vi "gnuplotVectors.vi"(4 "VectorFileLocation":path) -> (0 "Plot data file":path, 1 "gnuplotScript":string, 2 "Saved Automatically?":bool)   [LabVIEW 2013]
uses:
  Results_plotter_Global.vi
panel:
  in  "OpenLogfile?":bool
  in  "Show Script Editor?":bool
  in  "Tab Control":enum32{"OtherStuff ", "TerminalTest"}(tab)
  out "AuditTrail":string[](array[string])
  # "Shows the numbered line colours and point styles available- well it would, if it didn't disappear every time I update from the repository..!"
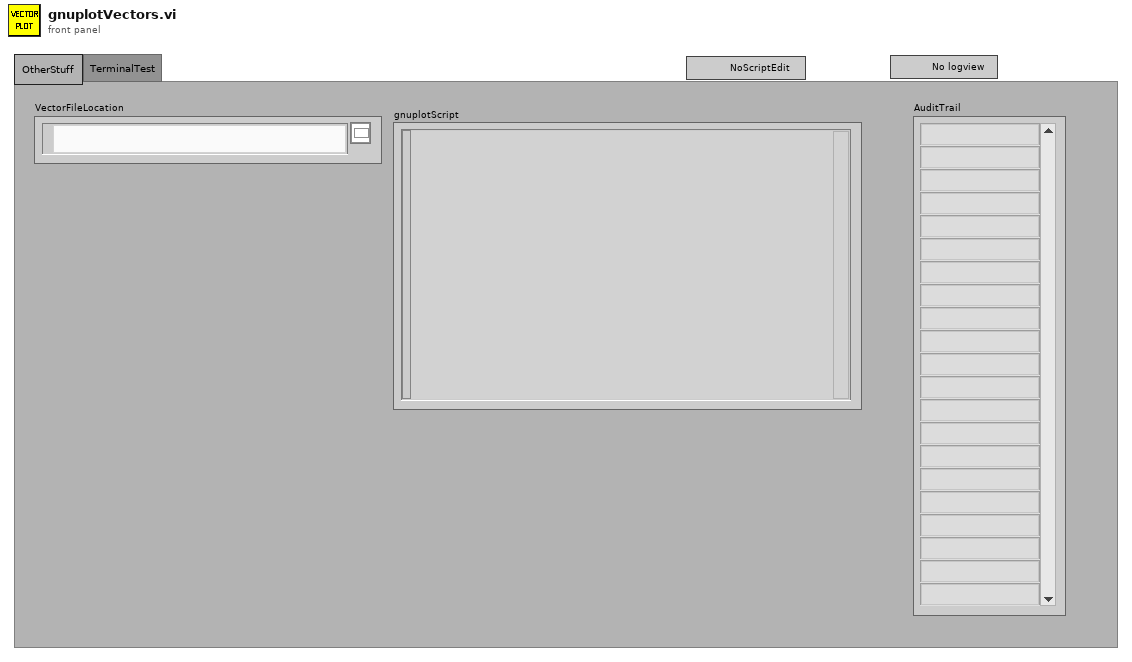
[diagram p1: front panel]
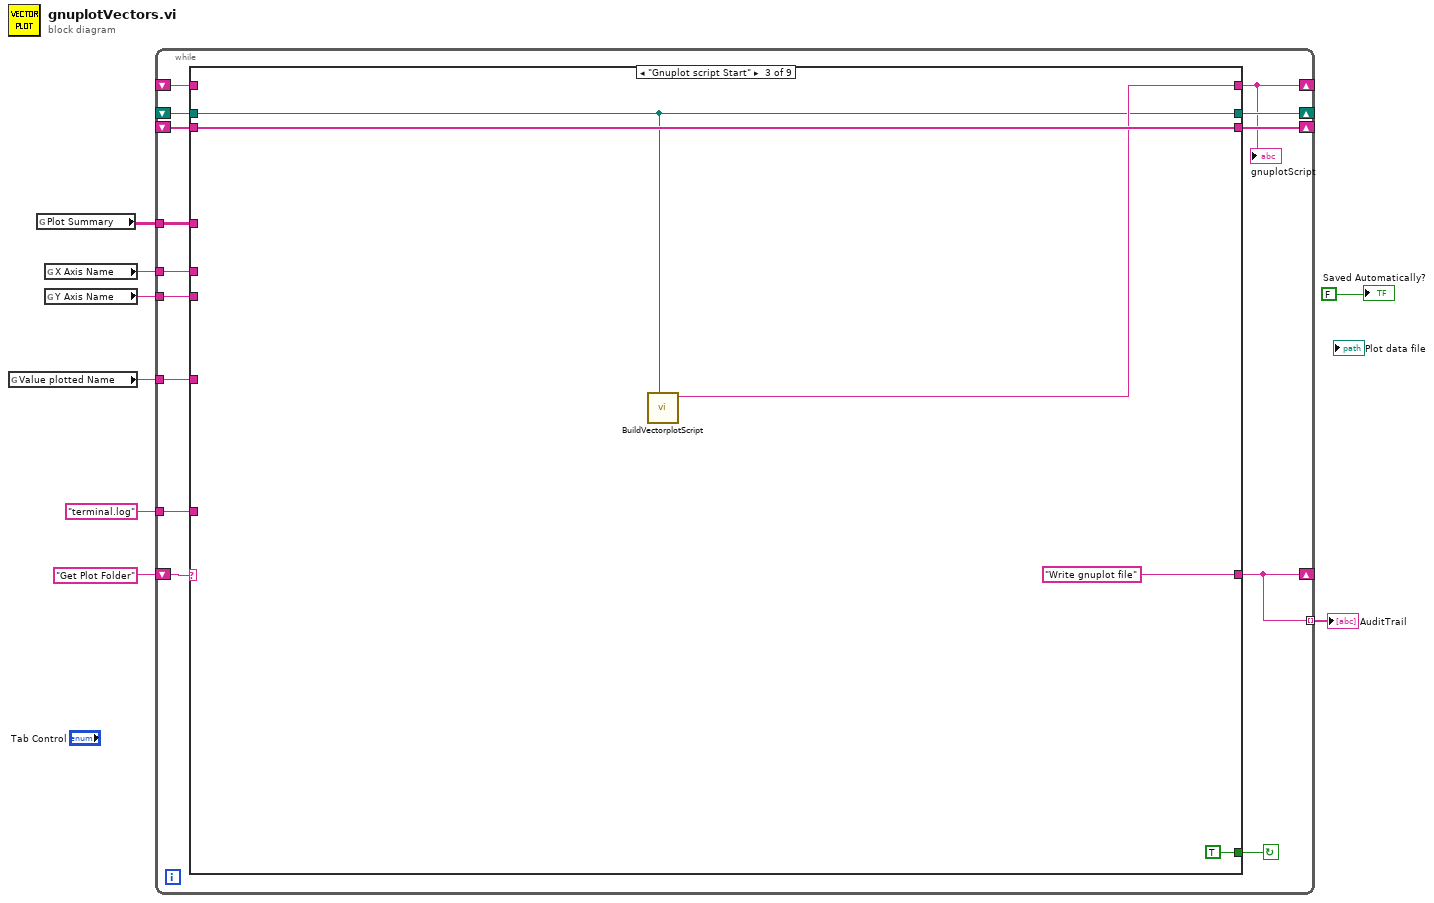
[diagram p0: block diagram]
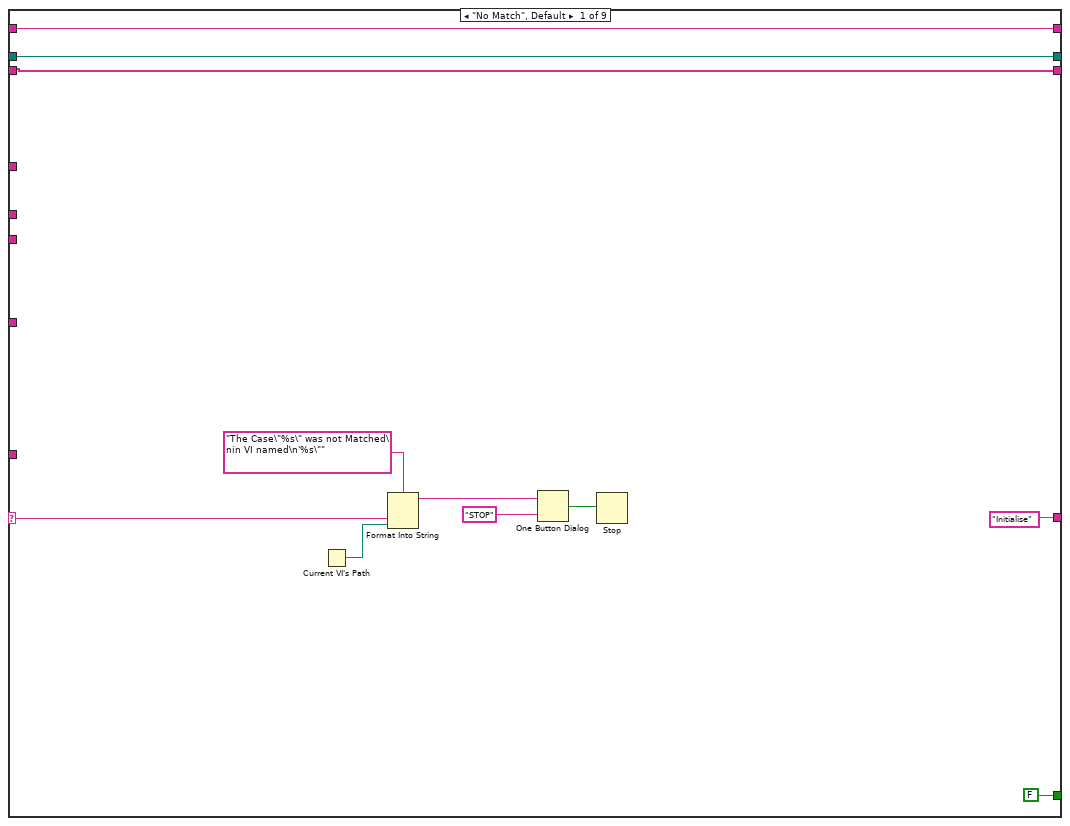
[diagram p2: hidden frame]
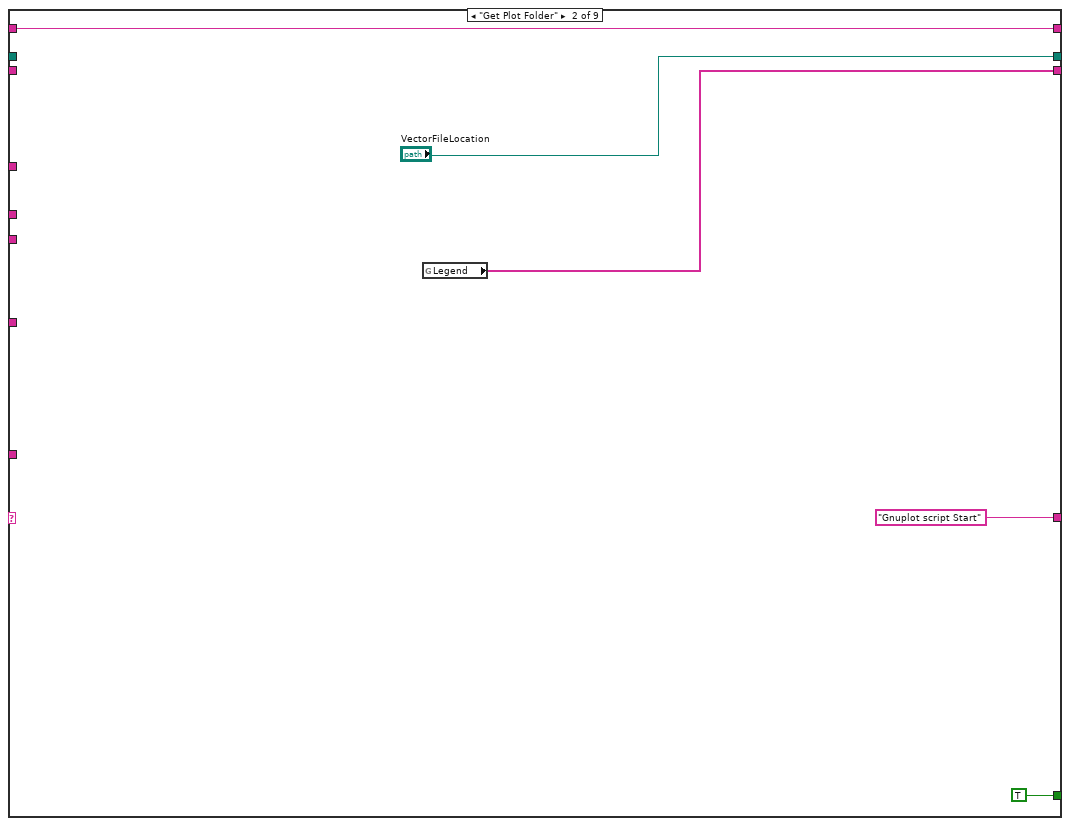
[diagram p3: hidden frame]
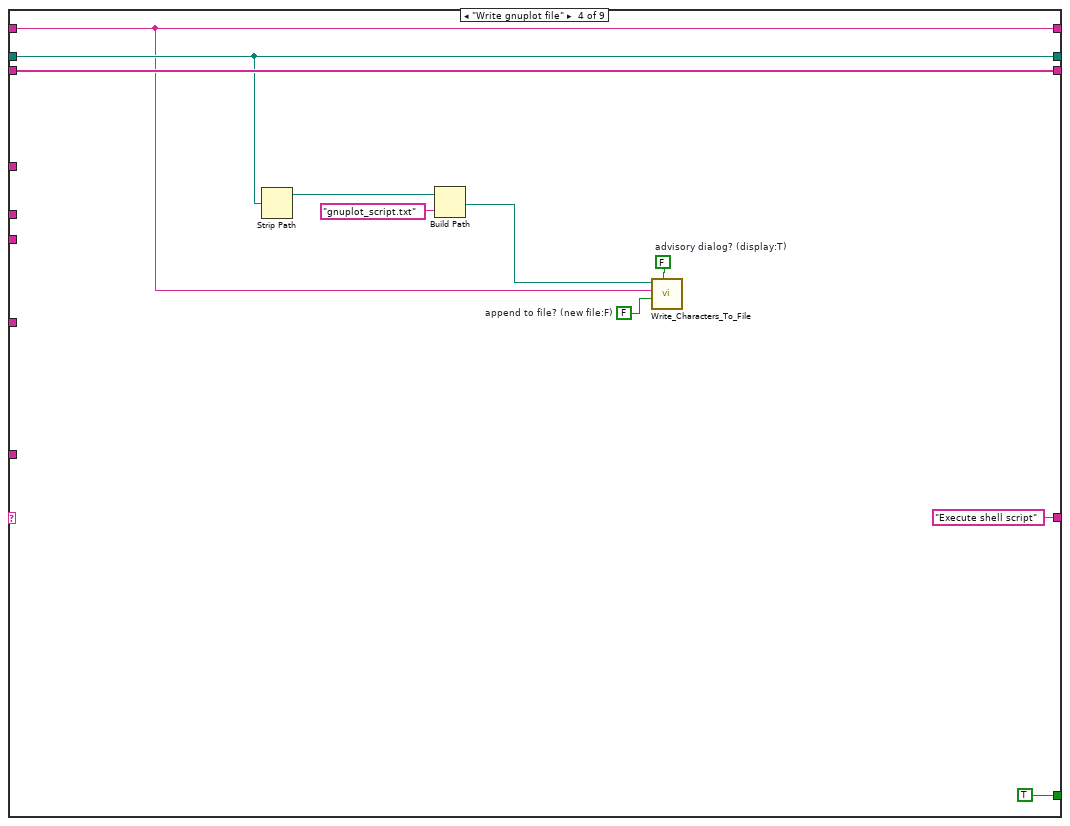
[diagram p4: hidden frame]
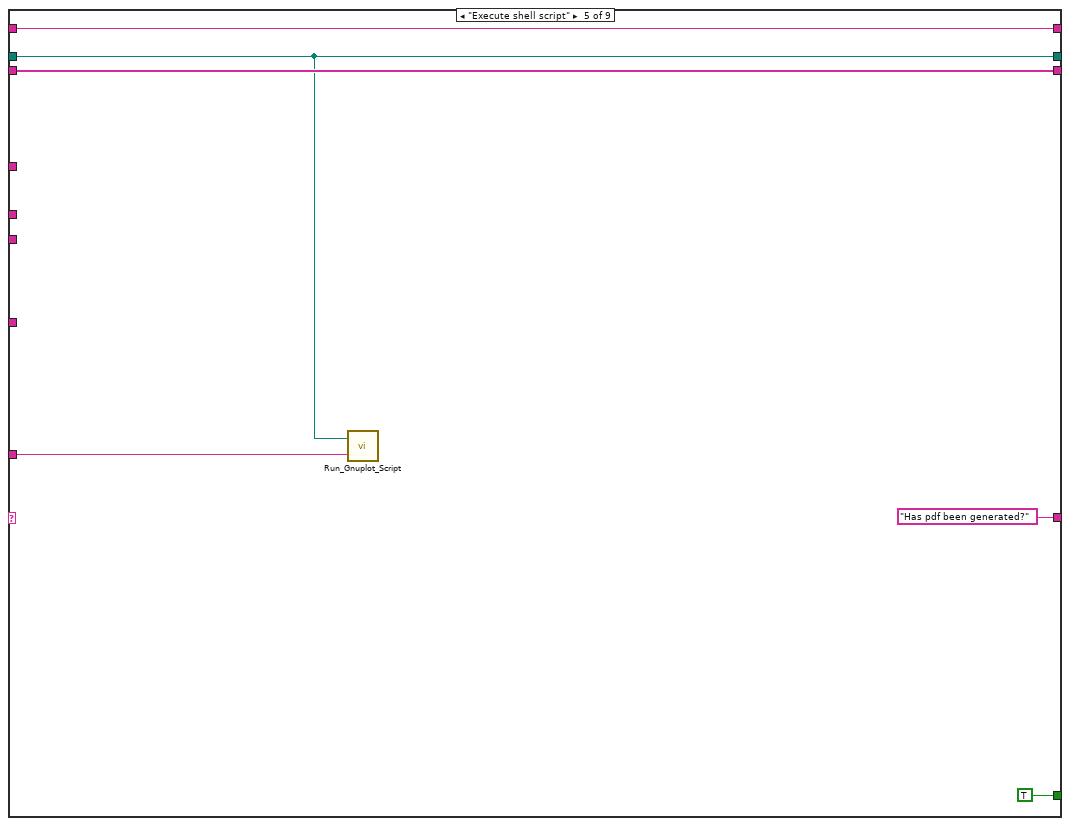
[diagram p5: hidden frame]
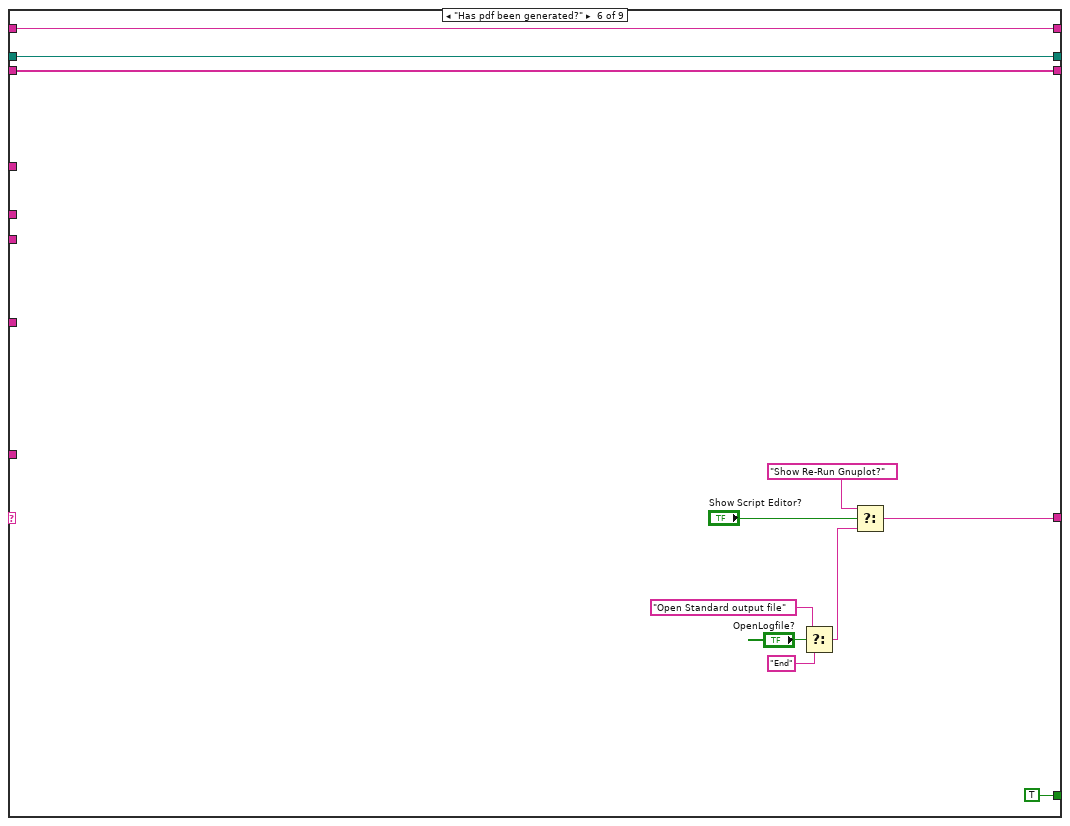
[diagram p6: hidden frame]
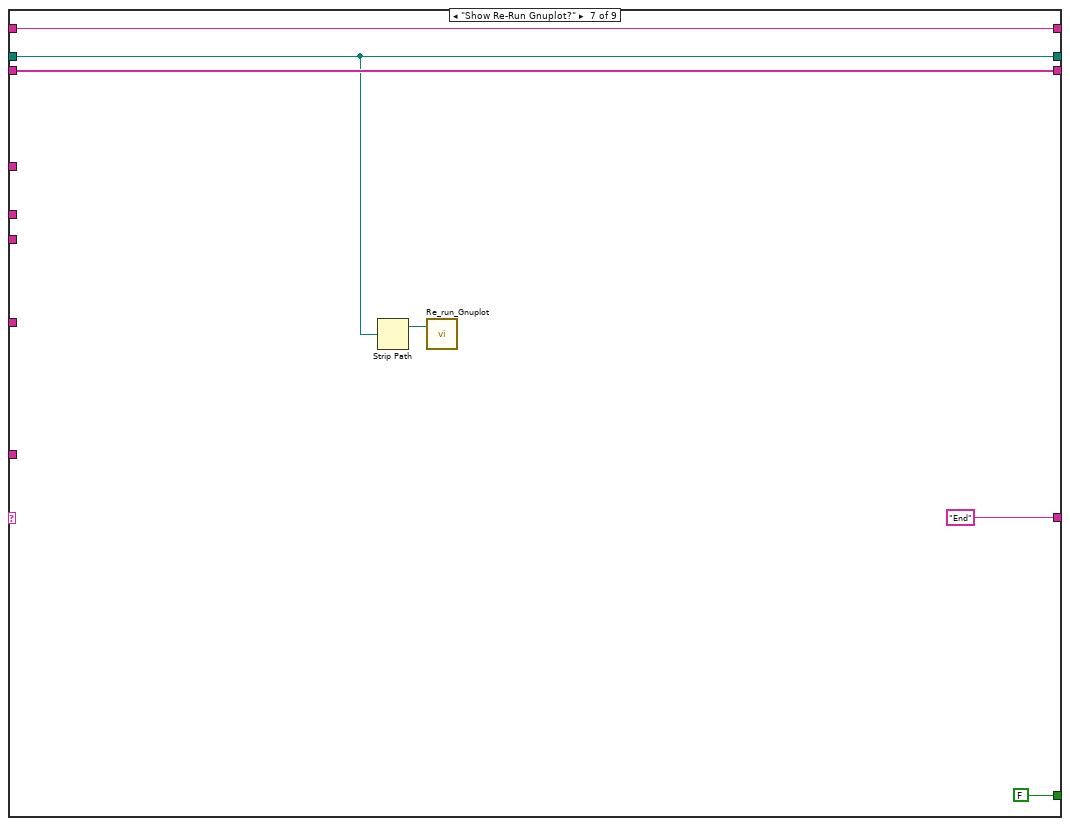
[diagram p7: hidden frame]
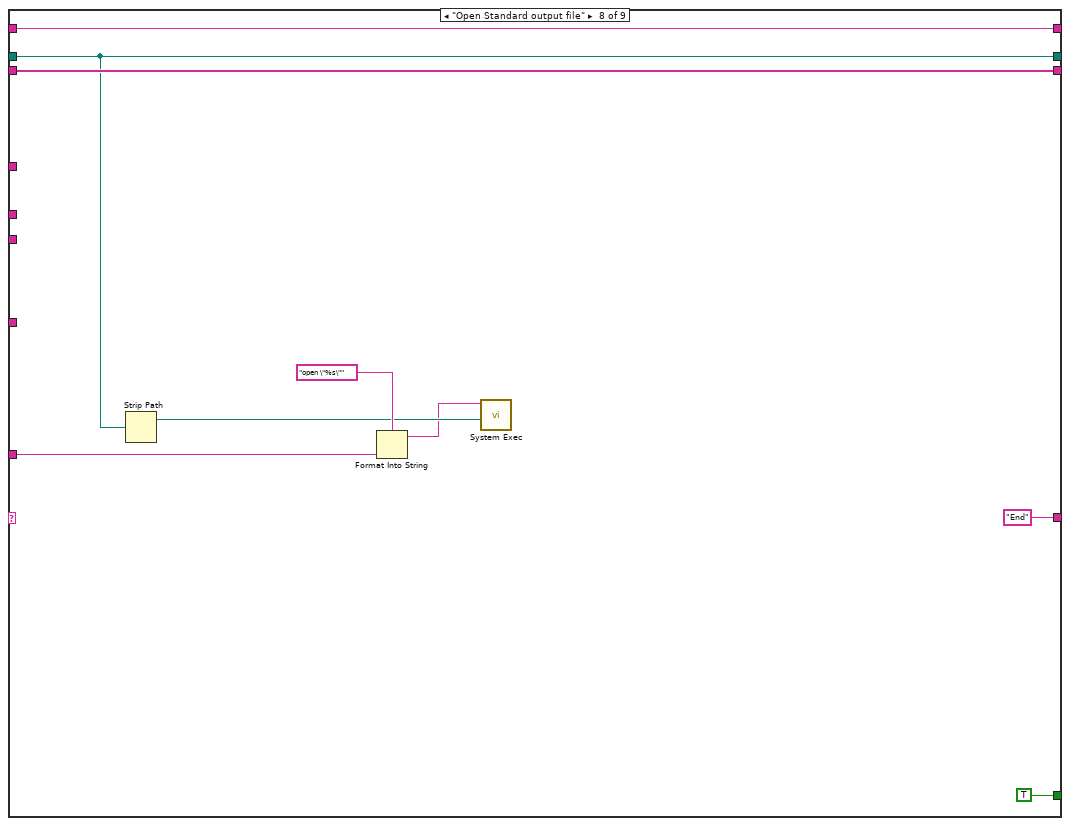
[diagram p8: hidden frame]
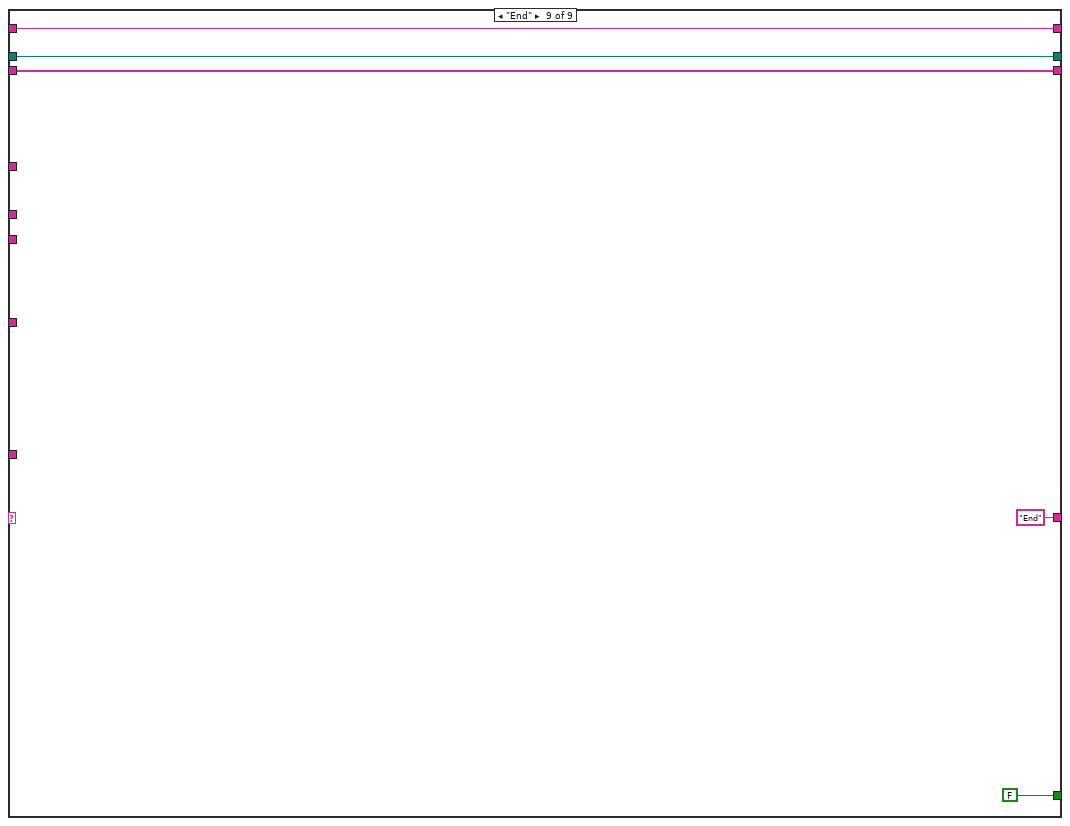
[diagram p9: hidden frame]
diagram:
  n1 = global read "Results_plotter_Global.vi" "Value plotted Name"() -> (w4:string)
  n2 = global read "Results_plotter_Global.vi" "Plot Summary"() -> (w7:string[][])
  n3 = global read "Results_plotter_Global.vi" "X Axis Name"() -> (w6:string)
  n4 = global read "Results_plotter_Global.vi" "Y Axis Name"() -> (w5:string)
  n5 = while {
    shift-left: "Get Plot Folder" -> [w21]
    shift-right: [w9] -> _
    tunnel: w7 -> [w20]
    shift-right: [w19] -> _
    shift-left: _ -> [w18]
    tunnel: w6 -> [w17]
    tunnel: w5 -> [w16]
    tunnel: w4 -> [w15]
    shift-right: [w10] -> _
    shift-left: _ -> [w14]
    shift-right: [w13] -> _
    shift-left: _ -> [w12]
    tunnel: "terminal.log" -> [w11]
    tunnel: [w9] -> w1 mode=indexing
    stop <- w22 continue-if-true
    n6 = case shown="\"Gnuplot script Start\"" w21 {
      selector: w21 -> [w23 _ _ _ _ _ _ _ _]
      tunnel: [FALSE TRUE TRUE ("Top Level") TRUE ("Top Level") TRUE ("Top Level") TRUE ("Top Level") FALSE ("Top Level") TRUE ("Top Level") FALSE ("Top Level")] -> w22
      tunnel: ["Initialise" "Gnuplot script Start" "Write gnuplot file" ("t") "Execute shell script" ("t") "Has pdf been generated?" ("t") w64 "End" "End" ("t") "End" ("t")] -> w9
      tunnel: w20 -> [_ _ _ _ _ _ _ _ _]
      tunnel: [w26 "VectorFileLocation" w39 w48 w55 w68 w72 w81 w90] -> w19
      tunnel: w18 -> [w26 _ w39 w48 w55 w68 w72 w81 w90]
      tunnel: w17 -> [_ _ _ _ _ _ _ _ _]
      tunnel: w16 -> [_ _ _ _ _ _ _ _ _]
      tunnel: w15 -> [_ _ _ _ _ _ _ _ _]
      tunnel: w14 -> [w25 w37 _ w44 w58 w69 w75 w84 w89]
      tunnel: [w25 w37 w40 w44 w58 w69 w75 w84 w89] -> w10
      tunnel: [w24 w36 w43 w49 w59 w70 w76 w85 w88] -> w13
      tunnel: w12 -> [w24 _ w43 w49 w59 w70 w76 w85 w88]
      tunnel: w11 -> [_ _ _ _ w54 _ _ w79 _]
      frame "No Match", Default {
        n7 = Current VI's Path() -> (path=w28:path)
        n8 = Format Into String(format string="The Case\"%s\" was not Matched\nin VI named\n'%s\"" ("Format String"), w23, w28) -> (resulting string=w31:string)  [unwired: 2 in, 1 out]
        n9 = One Button Dialog(message=w31, button name ("OK")="STOP") -> (true=w29:bool)
        n10 = Stop(stop? (T)=w29) -> ()
      }
      frame "Get Plot Folder" {
        n11 = global read "Results_plotter_Global.vi" "Legend"() -> (w36:string[])
      }
      frame "Gnuplot script Start" {
        n12 = call "BuildVectorplotScript.vi"("datafilePath"=w39) -> ("String out"=w40:string)  [unwired: 10 in]
      }
      frame "Write gnuplot file" {
        w51 = FALSE  # append to file? (new file:F)
        w52 = FALSE  # advisory dialog? (display:T)
        n13 = Strip Path(path=w48) -> (stripped path=w45:path)  [unwired: 1 out]
        n14 = Build Path(base path=w45, name or relative path="gnuplot_script.txt") -> (appended path=w53:path)
        n15 = call "Write_Characters_To_File.vi"("file path (dialog if empty)"=w53, "advisory dialog? (display:T)"=w52, "character string"=w44, "append to file? (new file:F)"=w51) -> ()  [unwired: 1 in, 4 out]
      }
      frame "Execute shell script" {
        n16 = call "Run_Gnuplot_Script.vi"("logfileName"=w54, "workingDirectory"=w55) -> ()
      }
      frame "Has pdf been generated?" {
        n17 = Select(t="Open Standard output file" ("f"), s="OpenLogfile?", f="End") -> (s? t:f=w60:string)
        n18 = Select(t="Show Re-Run Gnuplot?", s="Show Script Editor?", f=w60) -> (s? t:f=w64:string)
      }
      frame "Show Re-Run Gnuplot?" {
        n19 = Strip Path(path=w72) -> (stripped path=w71:path)  [unwired: 1 out]
        n20 = call "Re_run_Gnuplot.vi"("Plot folder (dialog if empty)"=w71) -> ()  [unwired: 4 out]
      }
      frame "Open Standard output file" {
        n21 = Strip Path(path=w81) -> (stripped path=w78:path)  [unwired: 1 out]
        n22 = Format Into String(format string="open \"%s\"", w79) -> (resulting string=w77:string)  [unwired: 2 in, 1 out]
        n23 = call <vilib>:"System Exec.vi"("working directory"=w78, "command line"=w77) -> ()  [unwired: 4 in, 6 out]
      }
      frame "End" {
      }
    }
    "gnuplotScript" <- w10
  }
  "AuditTrail" <- w1
  "Saved Automatically?" <- FALSE
